vi "SENS_FOM_RANG_FREQ_STOP.vi"(0 "VISA IN":refnum<visa-resource-name>, 1 "Range number":i32, 2 "Frq. Stop":dbl, 5 "error in":errorcluster, 7 "Channel":i32) -> (14 "VISA Out":refnum<visa-resource-name>, 19 "error out":errorcluster)   [LabVIEW 2018, in "PNA-X.lvlib"]
doc: "SENSe<cnum>:FOM:RANGe<n>:FREQuency:STOP <num> \n(Read-Write) Sets and returns the Stop value of frequency range. Also specify Start frequency. \nThis setting is valid for the primary range, or if the specified range is already uncoupled from the primary range \nand if the sweep type is LOG or LINear. \nParameters \n<cnum> Any existing channel number; if unspecified, value is set to 1. \n<n> Range number. If unspecified, value is set to 1. \n<num> Stop value in Hz. Choose any frequency within the range of the PNA. \nExamples SENS:FOM:RANG:FREQ:STOP 1e12 \nsense2:fom:range2:frequency:stop 10000000000 \nQuery Syntax SENSe<cnum>:FOM:RANGe<n>:FREQuency:STOP? \nReturn Type Numeric \nDefault Maximum frequency of the PNA."
uses:
  PNA-X.lvlib
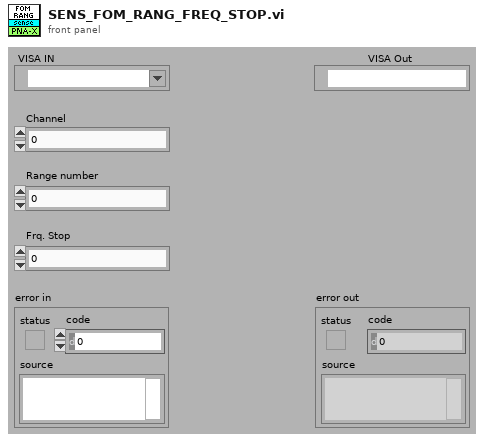
[diagram p1: front panel]
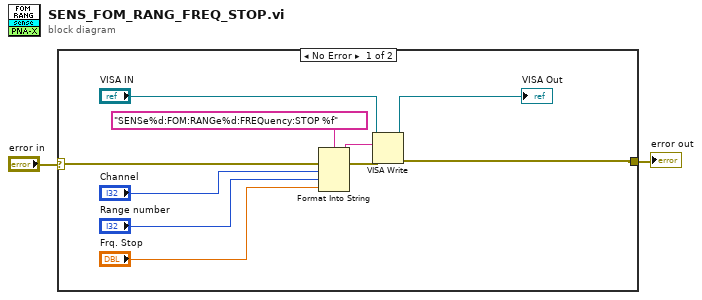
[diagram p0: block diagram]
diagram:
  n1 = case shown="No Error" "error in" {
    selector: "error in" -> [w12 w13]
    tunnel: [w7 w13] -> w1
    frame No Error {
      n2 = Format Into String(format string="SENSe%d:FOM:RANGe%d:FREQuency:STOP %f" ("Cmdline"), error in=w12, "Channel", "Range number", "Frq. Stop") -> (resulting string=w10:string, error out=w11:errorcluster)  [unwired: 1 in]
      n3 = VISA Write(VISA resource name="VISA IN", write buffer=w10, error in (no error)=w11) -> (VISA resource name out=→"VISA Out":refnum<visa-resource-name>, error out=w7:errorcluster)  [unwired: 1 out]
    }
    frame Error {
    }
  }
  "error out" <- w1
